vi "Orientation Approach Vectors to Rotation Matrix.vi"(1 "approach":dbl[](array[numeric]), 2 "orientation":dbl[](array[numeric])) -> (0 "rotation matrix":T1)   [LabVIEW 2017, in "NI_Kinematics.lvlib"]
uses:
  <vilib>/robotics/Kinematics/NI_Kinematics.lvlib
  <vilib>/Analysis/Matrix/Datatypes/RealMatrix.ctl
  <vilib>/Analysis/_algsub.llb/Real Vector Norm.vi
  <vilib>/Analysis/NI_AALPro.lvlib
  <vilib>/Analysis/Matrix/NI_Matrix.lvlib
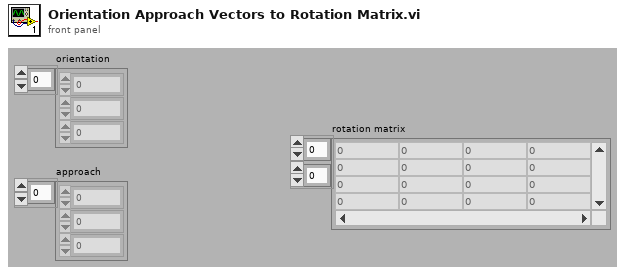
[diagram p1: front panel]
types:
  T1 = typedef "NI_Matrix.lvlib/RealMatrix.ctl" = dbl[][]
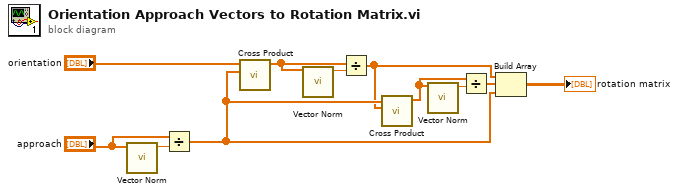
[diagram p0: block diagram]
diagram:
  n1 = call-poly <vilib>:"Vector Norm.vi"("Input Vector"="approach") -> ("norm"=w11:dbl)  [unwired: 9 in, 1 out]
  n2 = Divide(x="approach", y=w11) -> (x/y=w9:dbl[])
  n3 = call <vilib>:"Cross Product.vi"("B Vector"=w9, "A Vector"="orientation") -> ("Cross Product"=w6:dbl[])  [unwired: 8 in, 1 out]
  n4 = call-poly <vilib>:"Vector Norm.vi"("Input Vector"=w6) -> ("norm"=w7:dbl)  [unwired: 9 in, 1 out]
  n5 = Divide(x=w6, y=w7) -> (x/y=w1:dbl[])
  n6 = call <vilib>:"Cross Product.vi"("B Vector"=w1, "A Vector"=w9) -> ("Cross Product"=w4:dbl[])  [unwired: 8 in, 1 out]
  n7 = call-poly <vilib>:"Vector Norm.vi"("Input Vector"=w4) -> ("norm"=w5:dbl)  [unwired: 9 in, 1 out]
  n8 = Divide(x=w4, y=w5) -> (x/y=w3:dbl[])
  n9 = Build Array(w1, w3, w9) -> (→"rotation matrix":T1)
